vi "Translator Array Get Pointer.vi"(0 "Input":variant=variant("Function Name"=variant(string "Strip Path"), "Input Datatypes"=variant(string[] ["error", "int"]), "Inputs"=variant(string[] ["error in", "x"]), "Node refnum"=variant(refnum<vi> refnum), "Output Datatypes"=variant(string[] ["int"]), "Outputs"=variant(string[] ["a"])), 11 "error in (no error)":errorcluster) -> (4 "Output":variant=variant("Defines"=variant(string[] []), "Includes"=variant(string[] []), "Replaced Code"=variant(string "/* LabVIEW system function 'Strip Path' not found. */")), 15 "error out":errorcluster)   [LabVIEW 2014]
doc: "An example of how to create the Translator to convert the LabVIEW VIs to Arduino C code."
panel:
  out "Outputs":string[](array[string])
  out "Inputs":string[](array[string])
  out "Output Datatypes":string[](array[string])
  out "Input Datatypes":string[](array[string])
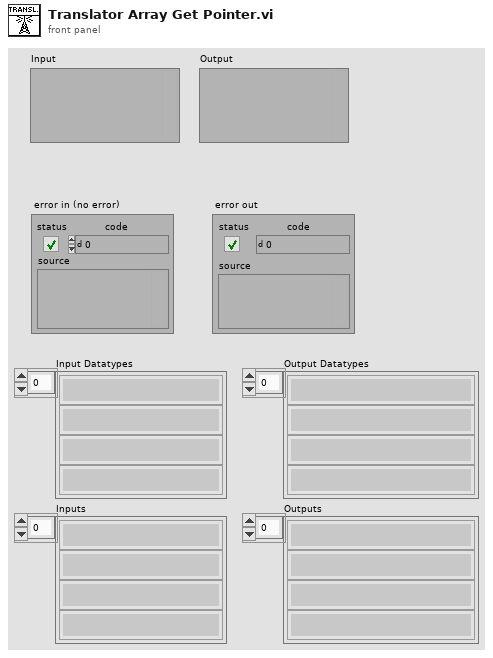
[diagram p1: front panel]
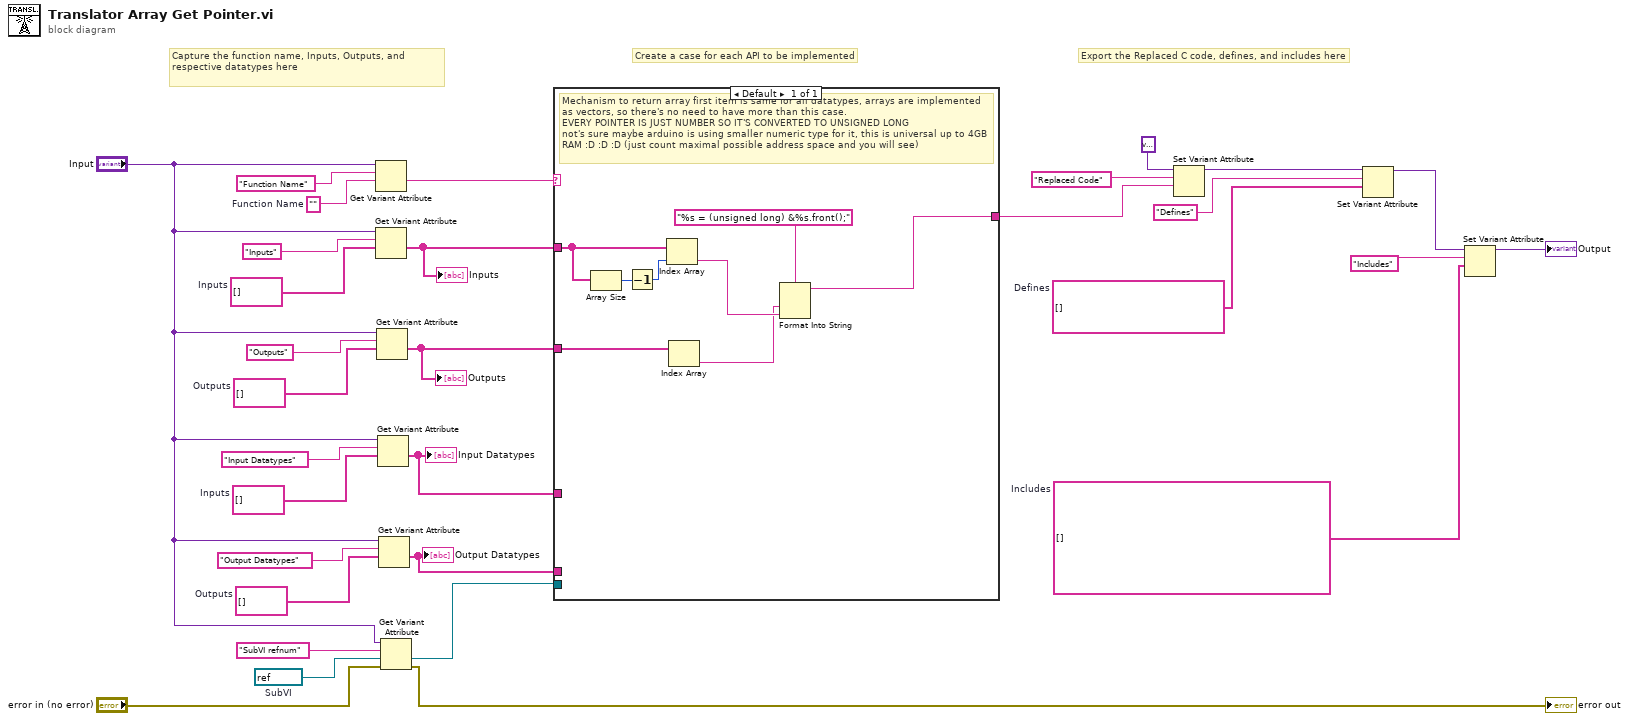
[diagram p0: block diagram]
diagram:
  w7 = refnum<vi> refnum  # SubVI
  w4 = string[] []  # Defines
  w17 = string[] []  # Outputs
  w18 = string[] []  # Inputs
  w3 = string[] []  # Includes
  w27 = string[] []  # Outputs
  w28 = string[] []  # Inputs
  w29 = ""  # Function Name
  # "Capture the function name, Inputs, Outputs, and respective datatypes here"
  # "Export the Replaced C code, defines, and includes here"
  # "Create a case for each API to be implemented"
  n1 = Get Variant Attribute(Variant="Input", name="Function Name", default value (empty Variant)=w29) -> (value=w24:string)  [unwired: 1 in, 3 out]
  n2 = Get Variant Attribute(Variant="Input", name="Inputs", default value (empty Variant)=w28) -> (value=w14:string[])  [unwired: 1 in, 3 out]
  "Inputs" <- w14
  n3 = Get Variant Attribute(Variant="Input", name="Outputs", default value (empty Variant)=w27) -> (value=w15:string[])  [unwired: 1 in, 3 out]
  "Outputs" <- w15
  n4 = Get Variant Attribute(Variant="Input", name="Input Datatypes", default value (empty Variant)=w18) -> (value=w10:string[])  [unwired: 1 in, 3 out]
  "Input Datatypes" <- w10
  n5 = Get Variant Attribute(Variant="Input", name="Output Datatypes", default value (empty Variant)=w17) -> (value=w5:string[])  [unwired: 1 in, 3 out]
  "Output Datatypes" <- w5
  n6 = Get Variant Attribute(Variant="Input", name="SubVI refnum", default value (empty Variant)=w7, error in="error in (no error)") -> (value=w6:refnum<vi>, error out=→"error out":errorcluster)  [unwired: 2 out]
  n7 = case shown="Default" w24 {
    tunnel: [w32] -> w23
    tunnel: w14 -> [w38]
    tunnel: w15 -> [w36]
    tunnel: w10 -> [_]
    tunnel: w6 -> [_]
    tunnel: w5 -> [_]
    frame Default {
      # "Mechanism to return array first item is same for all datatypes, arrays are implemented as vectors, so there's no need to have more than this case.\nEVERY POINTER IS JUST NUMBER SO IT'S CONVERTED TO UNSIGNED LONG\nnot's sure maybe arduino is using smaller numeric type for it, this is universal up to 4GB RAM :D :D :D (just count maximal possible address space and you will see)"
      n8 = Array Size(array=w38) -> (size(s)=w39:i32)
      n9 = Decrement(x=w39) -> (x-1=w37:i32)
      n10 = Index Array(array=w38, index=w37) -> (element=w34:string)
      n11 = Index Array(array=w36) -> (element=w33:string)  [unwired: 1 in]
      n12 = Format Into String(format string="%s = (unsigned long) &%s.front();", w33, w34) -> (resulting string=w32:string)  [unwired: 2 in, 1 out]
    }
  }
  n13 = Set Variant Attribute(Variant=variant ("variant"), name="Replaced Code", value=w23) -> (Variant out=w13:variant)  [unwired: 1 in, 2 out]
  n14 = Set Variant Attribute(Variant=w13, name="Defines", value=w4) -> (Variant out=w12:variant)  [unwired: 1 in, 2 out]
  n15 = Set Variant Attribute(Variant=w12, name="Includes", value=w3) -> (Variant out=→"Output":variant)  [unwired: 1 in, 2 out]
